vi "oa_TV Time Index Angle (NChan).vi"(0 "pulse positions":cluster{dbl[]}[](array[cluster]), 5 "angle intervals":cluster{dbl[]}[](array[cluster]), 7 "revulotion":i32[](array[numeric]), 9 "revulotion index":i32[](array[numeric]), 11 "error in (no error)":errorcluster) -> (4 "pulse positions":cluster{dbl[]}[](array[cluster]), 6 "angle":cluster{dbl[]}[](array[cluster]), 15 "error out":errorcluster)   [LabVIEW 2017, in "SoundVib_Torsional.lvlib"]
uses:
  <vilib>/addons/Sound and Vibration/Order Analysis/Torsional Vibration/SoundVib_Torsional.lvlib
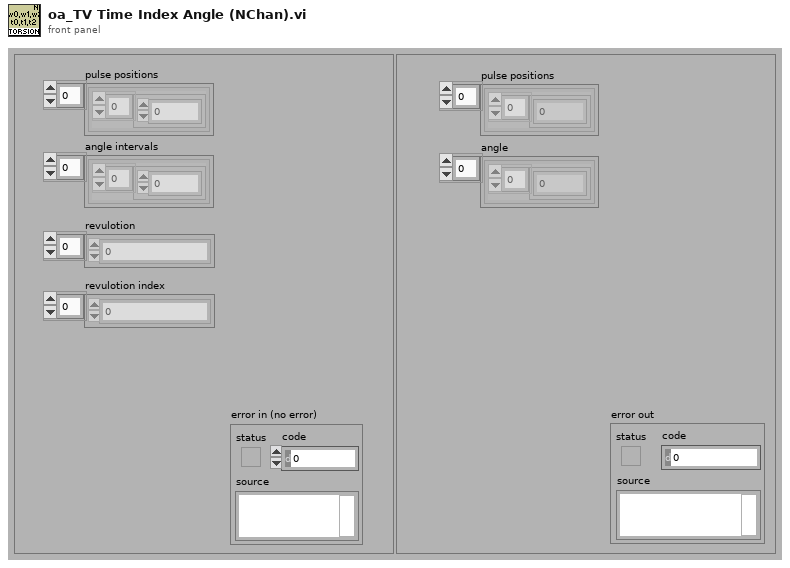
[diagram p1: front panel]
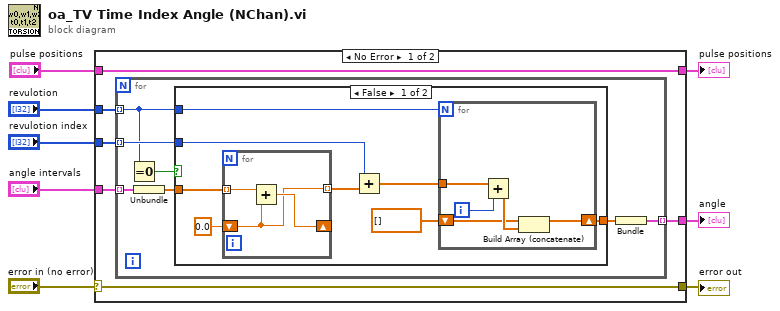
[diagram p0: block diagram]
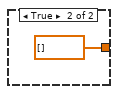
[diagram p2: hidden frame]
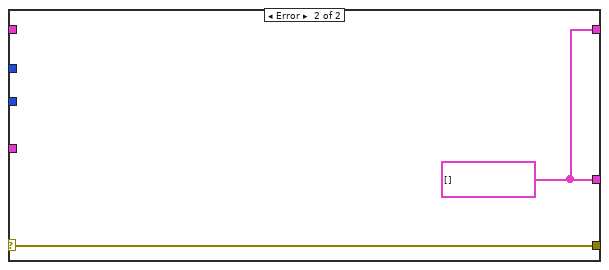
[diagram p3: hidden frame]
diagram:
  n1 = case shown="No Error" "error in (no error)" {
    selector: "error in (no error)" -> [w11 w40]
    tunnel: "angle intervals" -> [w14 _]
    tunnel: "revulotion index" -> [w13 _]
    tunnel: [w12 w39] -> w3
    tunnel: [w11 w40] -> w7
    tunnel: "revulotion" -> [w10 _]
    tunnel: "pulse positions" -> [w9 _]
    tunnel: [w9 w39] -> w1
    frame No Error {
      n2 = for {
        tunnel: w14 -> [w20] mode=indexing
        tunnel: w13 -> [w21] mode=indexing
        tunnel: [w17] -> w12 mode=indexing
        tunnel: w10 -> [w16] mode=indexing
        n3 = Equal To 0?(x=w16) -> (x = 0?=w15:bool)
        n4 = Unbundle(w20) -> (w19:dbl[])
        n5 = case shown="False" w15 {
          tunnel: w21 -> [w27 _]
          tunnel: w16 -> [w24 _]
          tunnel: w19 -> [w23 _]
          tunnel: [w22 dbl[] []] -> w18
          frame False {
            n6 = for {
              tunnel: w23 -> [w32] mode=indexing
              shift-right: [w31] -> _
              shift-left: 0.0 -> [w30]
              tunnel: [w30] -> w26 mode=indexing
              n7 = Add(x=w32, y=w30) -> (x+y=w31:dbl)
            }
            n8 = Add(x=w27, y=w26) -> (x+y=w25:dbl[])
            n9 = for {
              N: w24 -> [_]
              tunnel: w25 -> [w36]
              shift-right: [w34] -> w22
              shift-left: dbl[] [] -> [w33]
              i -> [w37]
              n10 = Add(x=w36, y=w37) -> (x+y=w35:dbl[])
              n11 = Build Array (concatenate)(w33, w35) -> (w34:dbl[])
            }
          }
          frame True {
          }
        }
        n12 = Bundle(w18) -> (w17:cluster{dbl[]})  [unwired: 1 in]
      }
    }
    frame Error {
      w39 = cluster{dbl[]}[] []
    }
  }
  "error out" <- w7
  "angle" <- w3
  "pulse positions" <- w1
